vi "micron_globals.vi"() -> ()   [LabVIEW 2014]
uses:
  testing/Micron params.ctl
  testing/stimulus.ctl
  testing/injection_point.ctl
  filtering/goal_loop_parms.ctl
  testing/mode_conrols.ctl
  testing/manipulator_cal.ctl
  asap/labview/testing/probe_calibration.ctl
  host/network_params.ctl
  cancellation/sq_control_params.ctl
  cancellation/decoupled_gain.ctl
  cancellation/estimation_controls.ctl
  micron_config.ctl
  manipulator/squiggle/Host/i2c_interface.ctl
  manipulator/squiggle/Host/fpga_reference.ctl
  asap/labview/initialization/configuration.ctl
  asap/labview/initialization/asap_calibration.ctl
  <vilib>/Analysis/Matrix/Datatypes/RealMatrix.ctl
  testing/log_event.ctl
  <vilib>/Analysis/Matrix/NI_Matrix.lvlib
panel:
  in  "Bad stimulus counter":i32
  out "Current status":T1[](array[typedef]) {"Timestamp" format="%<%.3X>T"}
  out "ASAP Config":T2
  in  "Axis scan":cluster{"Driven axis":i32, "Scan index":i32}
  out "Trace data magic":sgl=123.125 min=1 step=0.1 format="%#_8f"
  in  "Trace data version":sgl=1.3 min=1 step=0.1 format="%#_6f"
  out "Micron config":T5
  out "Parameters initialized":bool
  in  "Config path":path=path "C:/config"
  in  "Stimulate error point":T8
  in  "Simulate error counter":i32
  in  "Parameters":T9={"Stimulus"={"Type"=enum."Step", "Phase"=0.0, "Amplitude"=[0.0, 200.0, 0.0, 0.0, 0.0, 0.0], "Injection point"=enum."Total pose", "Closed loop"=TRUE, "Offset"=[0.0, 0.0, 0.0, 0.0, 0.0, 0.0], "Tip -> world"=TRUE, "Frequency"=1.0, "Length"=1.0}, "Goal Filter A"={"Speedup max"=100.0, "Speedup thresh"=1500.0, "Speedup nonlin"=2.0, "Filters"=[{"Lower Fc"=0.05, "Lower Q"=0.62, "Scale factor"=3.0, "Upper Fc"=2.0, "Upper Q"=0.62, "V limit"=1000.0, "V limit range"=1000.0}, {"Lower Fc"=0.05, "Lower Q"=0.62, "Scale factor"=3.0, "Upper Fc"=2.0, "Upper Q"=0.62, "V limit"=1000.0, "V limit range"=1000.0}]}, "Mode controls"={"Hold"=FALSE, "Cancellation"=FALSE, "Goal filter"=TRUE, "Trigger"=FALSE}, "Manipulator type"=enum."Current piezo", "Manipulator calibration"={"Tool offsets"=[[0.0, 0.0, 51250.0, 0.0, 0.0, 0.0], [0.0, 0.0, 10000.0, 0.0, 0.0, 0.0], [0.0, 0.0, 0.0, 0.0, 0.0, 36200.0]], "Handle light calibration"=[[8328.325, -13809.074, -27020.809], [789.8538, -13828.106, -39014.85], [-7177.4033, -14258.012, -27375.71]], "Base pivots"=[[2000.0, 9798.0, -28635.0], [-2000.0, 9798.0, -28635.0], [-9485.0, -3167.0, -28635.0], [-7485.0, -6631.0, -28635.0], [7485.0, -6631.0, -28635.0], [9485.0, -3167.0, -28635.0]], "Output pivots"=[[4810.0, 5086.0, -6135.0], [-4810.0, 5086.0, -6135.0], [-6810.0, 1622.0, -6135.0], [-2000.0, -6708.0, -6135.0], [2000.0, -6708.0, -6135.0], [6810.0, 1622.0, -6135.0]], "Length center"=23200.0, "Workspace height"=[4000.0, 20000.0], "Workspace diameter"=[4000.0, 4000.0, 0.0, 0.0, 36200.0], "Stack travel"=2650.0, "Saturation pos"=2300.0, "Inverse filters"=[{"filter structure"=enum."IIR 2nd Order", "Reverse Coefficients"=[0.0, 0.0], "Forward Coefficients"=[1.0, 0.0, 0.0]}, {"filter structure"=enum."IIR 2nd Order", "Reverse Coefficients"=[0.0, 0.0], "Forward Coefficients"=[1.0, 0.0, 0.0]}, {"filter structure"=enum."IIR 2nd Order", "Reverse Coefficients"=[0.0, 0.0], "Forward Coefficients"=[1.0, 0.0, 0.0]}, {"filter structure"=enum."IIR 2nd Order", "Reverse Coefficients"=[0.0, 0.0], "Forward Coefficients"=[1.0, 0.0, 0.0]}], "Strut length"=10000.0, "Tip light calibration"=[[-1304.3153, -14438.996, -12817.332], [773.9923, -14294.808, -22046.66], [2960.8306, -14418.478, -12768.43]]}, "Network"={"Remote Host"="192.168.1.14", "Send Status"=TRUE, "Send Port"=61557, "Recv Commands"=TRUE, "Recv Port"=61558}, "Goal Filter B"={"Speedup max"=10.0, "Speedup thresh"=750.0, "Speedup nonlin"=2.0, "Filters"=[{"Lower Fc"=1.5, "Lower Q"=0.62, "Scale factor"=1.0, "Upper Fc"=1.5, "Upper Q"=0.62, "V limit"=1000.0, "V limit range"=0.0}, {"Lower Fc"=1.5, "Lower Q"=0.62, "Scale factor"=1.0, "Upper Fc"=1.5, "Upper Q"=0.62, "V limit"=1000.0, "V limit range"=0.0}]}, "Cancellation"={"KP"={"XY"=0.5, "Rxy"=0.5, "Z"=0.2, "Rz"=0.1}, "KI"=0.0, "KD"={"XY"=-0.2, "Rxy"=0.0, "Z"=0.0, "Rz"=0.0}, "Max vel"=13.0, "Max acc"=2.0, "Int error limit"=3.0, "RCM gain"=1.0, "Bypass"=FALSE, "Degraded gain"=0.4}, "Transition time"=1.0, "Estimation"={"Link"={"Measure noise"=[4.0], "Process noise"=[15.0, 1.0], "Alt process noise"=[20.0], "Alt turnoff cycles"=20, "Innovation limit"=[inf], "Residue threshold"=20.0, "Enable"=TRUE}, "Handle"={"Measure noise"=[3.6, 0.00036], "Process noise"=[0.0, 0.0, 0.3, 0.0, 0.0006, 0.3, 1.0, 0.3, 0.3, 1.0], "State limits"=[], "Innovation limit"=[], "Prediction Lookahead"=1.5, "Enable"=TRUE}}} {"Transition time" format="%_3f"; "Cancellation"."Degraded gain" min=0 max=1 step=0.1 format="%#_3p"; "Cancellation"."RCM gain" min=0 max=1 step=0.1 format="%#_3p"; "Cancellation"."KD"."Rz" min=-1 max=1 step=0.01 format="%#_3p"; "Cancellation"."KD"."Rxy" min=-1 max=1 step=0.01 format="%#_3p"; "Cancellation"."KD"."Z" min=-1 max=1 step=0.01 format="%#_3p"; "Cancellation"."KD"."XY" min=-1 max=1 step=0.01 format="%#_3p"; "Cancellation"."KI" min=0 max=1 step=0.01 format="%#_3p"; "Cancellation"."KP"."Rz" min=-1 max=1 step=0.01 format="%#_3p"; "Cancellation"."KP"."Rxy" min=-1 max=1 step=0.01 format="%#_3p"; "Cancellation"."KP"."Z" min=-1 max=1 step=0.01 format="%#_3p"; "Cancellation"."KP"."XY" min=-1 max=1 step=0.01 format="%#_3p"; "Cancellation"."Max acc" format="%#_3p"; "Goal Filter B"."Filters"."V limit range" format="%_3p"; "Goal Filter B"."Filters"."V limit" format="%_3p"; "Goal Filter B"."Filters"."Upper Q" format="%_3f"; "Goal Filter B"."Filters"."Upper Fc" format="%_3p"; "Goal Filter B"."Filters"."Lower Q" format="%_3f"; "Goal Filter B"."Filters"."Scale factor" format="%_3f"; "Goal Filter B"."Filters"."Lower Fc" format="%_3p"; "Goal Filter B"."Speedup nonlin" format="%_3p"; "Goal Filter B"."Speedup thresh" format="%_3p"; "Goal Filter B"."Speedup max" format="%_3p"; "Manipulator calibration"."Tip light calibration" format="%#.1f"; "Manipulator calibration"."Strut length" format="%#_4p"; "Manipulator calibration"."Saturation pos" format="%#.1f"; "Manipulator calibration"."Stack travel" format="%#.1f"; "Manipulator calibration"."Length center" format="%#_4p"; "Manipulator calibration"."Output pivots" format="%#_6f"; "Manipulator calibration"."Base pivots" format="%#_6f"; "Manipulator calibration"."Handle light calibration" format="%#.1f"; "Goal Filter A"."Filters"."V limit range" format="%_3p"; "Goal Filter A"."Filters"."V limit" format="%_3p"; "Goal Filter A"."Filters"."Upper Q" format="%_3f"; "Goal Filter A"."Filters"."Upper Fc" format="%_3p"; "Goal Filter A"."Filters"."Lower Q" format="%_3f"; "Goal Filter A"."Filters"."Scale factor" format="%_3f"; "Goal Filter A"."Filters"."Lower Fc" format="%_3p"; "Goal Filter A"."Speedup nonlin" format="%_3p"; "Goal Filter A"."Speedup thresh" format="%_3p"; "Goal Filter A"."Speedup max" format="%_3p"; "Stimulus"."Length" min=0.0 max=100.0 step=100.0 format="%#_4p"; "Stimulus"."Frequency" min=0.0 step=100.0 format="%#_4g"; "Stimulus"."Offset" format="%#_3p"; "Stimulus"."Amplitude" format="%#_3p"; "Stimulus"."Phase" min=-180.0 max=360.0 step=100.0 format="%#.2f"}
  # "Axis being driven in stimulus, 0..5"
  # "Sequence number in the scan series."
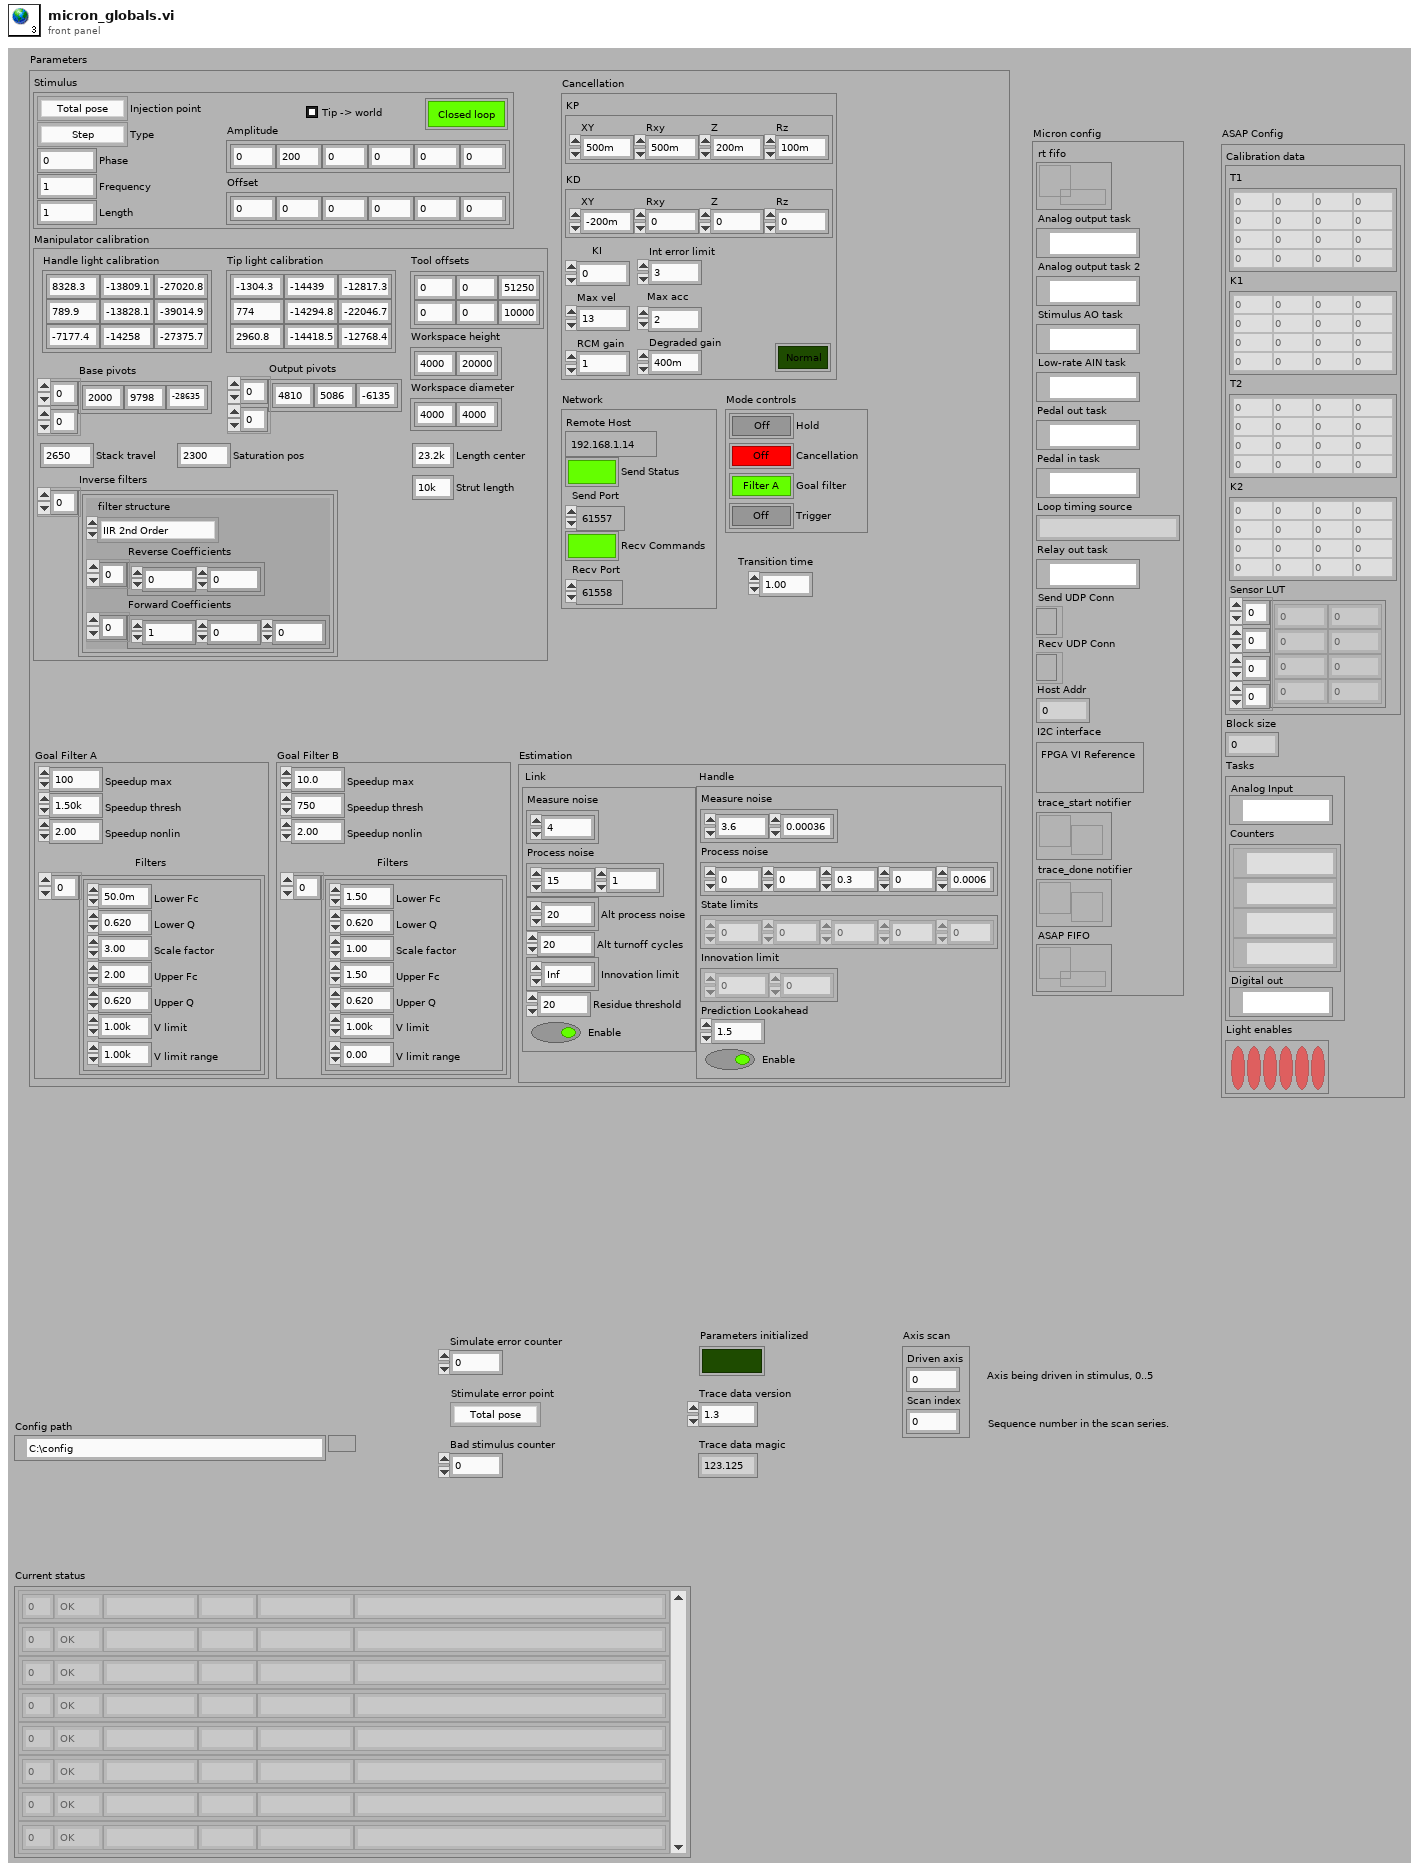
[diagram p1: front panel]
types:
  T1 = typedef "log_event.ctl" = cluster{"Facility ID":i32, "Severity":enum16{"OK", "Debug", "Warn", "Error"}, "Timestamp":timestamp, "Facility":string, "State":string, "Message":string}
  T2 = typedef "configuration.ctl" = cluster{"Calibration data":T3, "Block size":i32, "Tasks":cluster{"Analog Input":refnum<k21>, "Counters":refnum<k21>[], "Digital out":refnum<k21>}, "Light enables":bool[]}
  T3 = typedef "asap_calibration.ctl" = cluster{"T1":T4, "K1":T4, "T2":T4, "K2":T4, "Sensor LUT":sgl[][][][]}
  T4 = typedef "NI_Matrix.lvlib/RealMatrix.ctl" = dbl[][]
  T5 = typedef "micron_config.ctl" = cluster{"rt fifo":refnum<k33>, "Analog output task":refnum<k21>, "Analog output task 2":refnum<k21>, "Stimulus AO task":refnum<k21>, "Low-rate AIN task":refnum<k21>, "Pedal out task":refnum<k21>, "Pedal in task":refnum<k21>, "Loop timing source":string, "Relay out task":refnum<k21>, "Send UDP Conn":refnum<k16>, "Recv UDP Conn":refnum<k16>, "Host Addr":u32, "I2C interface":T6, "trace_start notifier":refnum<notifier>, "trace_done notifier":refnum<notifier>, "ASAP FIFO":refnum<k33>}
  T6 = typedef "i2c_interface.ctl" = cluster{"FPGA VI Reference":T7}
  T7 = typedef "fpga_reference.ctl" = refnum<k20>
  T8 = typedef "injection_point.ctl" = enum16{"Total pose", "V limiter", "Goal ", "Link position", "KF link position", "Inverse kin", "Link goal", "Link error", "Controller", "Output", "Drive", "Light"}
  T9 = typedef "Micron params.ctl" = cluster{"Stimulus":T10, "Goal Filter A":T11, "Mode controls":T12, "Manipulator type":enum16{"Current piezo", "Voltage piezo"}, "Manipulator calibration":T13, "Network":T15, "Goal Filter B":T11, "Cancellation":T16, "Transition time":sgl, "Estimation":T18}
  T10 = typedef "stimulus.ctl" = cluster{"Type":enum16{"Off", "Step", "Sine", "Triangle", "Arbitrary"}, "Phase":dbl, "Amplitude":sgl[], "Injection point":T8, "Closed loop":bool, "Offset":sgl[], "Tip -> world":bool, "Frequency":dbl, "Length":dbl}
  T11 = typedef "goal_loop_parms.ctl" = cluster{"Speedup max":sgl, "Speedup thresh":sgl, "Speedup nonlin":sgl, "Filters":cluster{"Lower Fc":sgl, "Lower Q":sgl, "Scale factor":sgl, "Upper Fc":sgl, "Upper Q":sgl, "V limit":sgl, "V limit range":sgl}[]}
  T12 = typedef "mode_conrols.ctl" = cluster{"Hold":bool, "Cancellation":bool, "Goal filter":bool, "Trigger":bool}
  T13 = typedef "manipulator_cal.ctl" = cluster{"Tool offsets":sgl[][], "Handle light calibration":T14, "Base pivots":sgl[][], "Output pivots":sgl[][], "Length center":sgl, "Workspace height":sgl[], "Workspace diameter":sgl[], "Stack travel":sgl, "Saturation pos":sgl, "Inverse filters":cluster{"filter structure":enum32{"IIR 2nd Order", "IIR 4th Order"}, "Reverse Coefficients":dbl[], "Forward Coefficients":dbl[]}[], "Strut length":sgl, "Tip light calibration":T14}
  T14 = typedef "probe_calibration.ctl" = sgl[][]
  T15 = typedef "network_params.ctl" = cluster{"Remote Host":string, "Send Status":bool, "Send Port":u16, "Recv Commands":bool, "Recv Port":u16}
  T16 = typedef "sq_control_params.ctl" = cluster{"KP":T17, "KI":sgl, "KD":T17, "Max vel":sgl, "Max acc":sgl, "Int error limit":sgl, "RCM gain":sgl, "Bypass":bool, "Degraded gain":sgl}
  T17 = typedef "decoupled_gain.ctl" = cluster{"XY":sgl, "Rxy":sgl, "Z":sgl, "Rz":sgl}
  T18 = typedef "estimation_controls.ctl" = cluster{"Link":cluster{"Measure noise":dbl[], "Process noise":dbl[], "Alt process noise":dbl[], "Alt turnoff cycles":i32, "Innovation limit":dbl[], "Residue threshold":dbl, "Enable":bool}, "Handle":cluster{"Measure noise":dbl[], "Process noise":dbl[], "State limits":dbl[], "Innovation limit":dbl[], "Prediction Lookahead":sgl, "Enable":bool}}
diagram:
